vi "osq_load.vi"(8 "error in (no error)":errorcluster, 11 "Open":path=path "C:/Users/Adam/Desktop/test.osq") -> (0 "error out":errorcluster, 2 "SEQs":T1[](array[typedef]), 3 "XML File Path(duplicate)":path, 4 "Lines":i32)   [LabVIEW 2015, in "oskar_tools.lvlib"]
uses:
  oskar_tools.lvlib
  seq_line.ctl
  <vilib>/Utility/xml.llb/Read From XML File(string).vi
panel:
  out "XML Elements":string
  in  "Template":T1[](array[typedef])
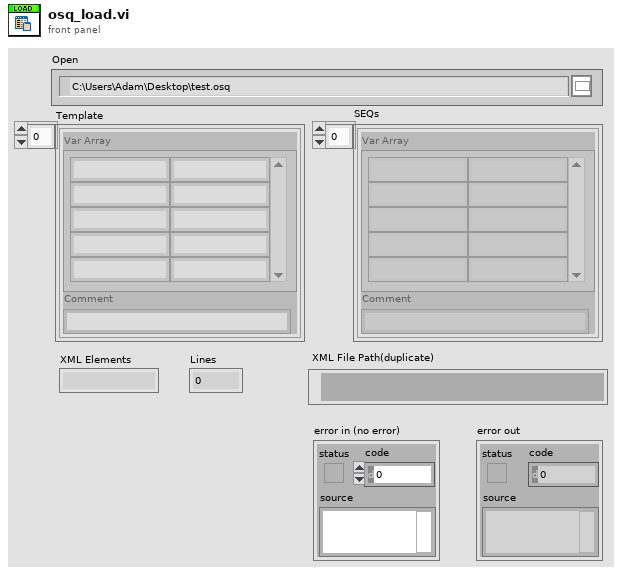
[diagram p1: front panel]
types:
  T1 = typedef "oskar_tools.lvlib/seq_line.ctl" = cluster{"Var Array":string[][], "Comment":string}
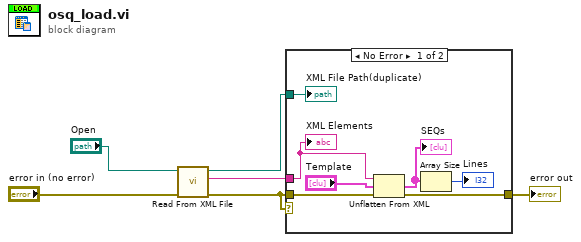
[diagram p0: block diagram]
diagram:
  n1 = call-poly <vilib>:"Read From XML File.vi"("error in (no error)"="error in (no error)", "XML File Path"="Open") -> ("error out"=w2:errorcluster, "XML Elements"=w3:string, "XML File Path(duplicate)"=w4:path)  [unwired: 7 in]
  n2 = case shown="No Error" w2 {
    tunnel: w4 -> [w13 _]
    tunnel: w3 -> [w10 _]
    tunnel: w2 -> [w11 w14]
    tunnel: [w9 w14] -> w1
    frame No Error {
      n3 = Unflatten From XML(xml string=w10, type="Template", error in (no error)=w11) -> (value=w8:T1[], error out=w9:errorcluster)
      "SEQs" <- w8
      n4 = Array Size(array=w8) -> (size(s)=→"Lines":i32)
      "XML File Path(duplicate)" <- w13
      "XML Elements" <- w10
    }
    frame Error {
    }
  }
  "error out" <- w1
